vi "Pickering7.vi"(3 "Xmit Ring":i8=1) -> (0 "error out":errorcluster, 2 "dup VISA resource name":refnum<visa-resource-name>)   [LabVIEW 2022 SP3]
uses:
  Motion Controllers/-MotionRoutines/MotionGlobals.vi
panel:
  # "A zero clears all switches. 1-5 selects Xmit ring"
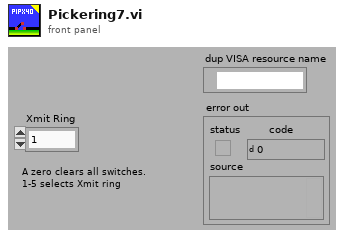
[diagram p1: front panel]
types:
  T1 = typedef "location.ctl" = enum16{"Automatic", "WCM Main", "Hawaii", "Columbia MM3000", "Columbia  NI System", "NYU", "RRI 2", "UHI Allen", "CUMC RT", "Chiba", "Stony Brook", "WCM Microscopy", "WCM Aeoretch", "WCM Optics Lab", "WCM Main 2Axis", "WCM Rotation", "WCM SAM SMAC", "SERI GP"}
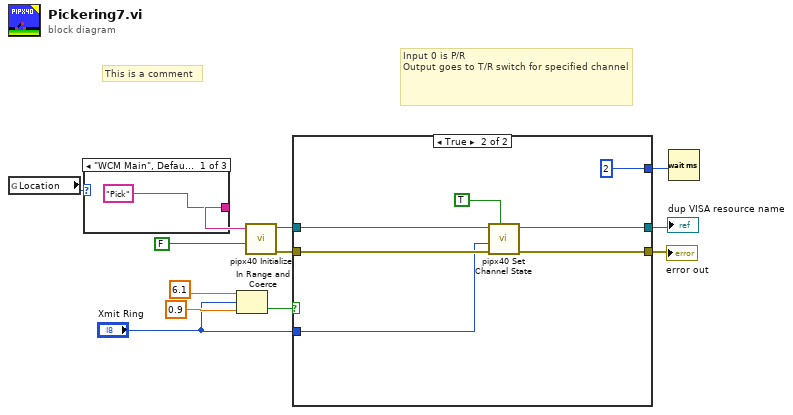
[diagram p0: block diagram]
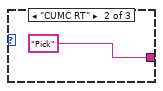
[diagram p2: hidden frame]
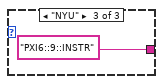
[diagram p3: hidden frame]
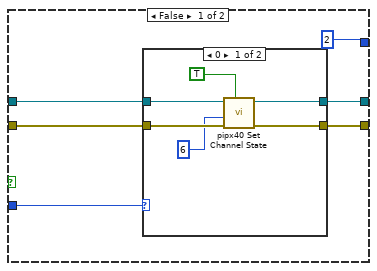
[diagram p4: hidden frame]
diagram:
  # "This is a comment"
  # "Input 0 is P/R\nOutput goes to T/R switch for specified channel"
  n1 = global read "MotionGlobals.vi" "Location"() -> (w2:T1)
  n2 = case shown="\"WCM Main\", Default" w2 {
    tunnel: ["Pick" ("VISA Resource Name") "Pick" ("VISA Resource Name") "PXI6::9::INSTR" ("VISA Resource Name")] -> w1
    frame "WCM Main", Default {
    }
    frame "CUMC RT" {
    }
    frame "NYU" {
    }
  }
  n3 = In Range and Coerce(upper limit=6.1, x="Xmit Ring", lower limit=0.9) -> (In Range?=w10:bool)  [unwired: 1 out]
  n4 = call <instrlib>:"pipx40 Initialize.vi"("reset device"=FALSE, "resource name"=w1) -> ("error out"=w5:errorcluster, "instrument handle out"=w6:refnum<visa-resource-name>)  [unwired: 8 in]
  n5 = case shown="True" w10 {
    tunnel: "Xmit Ring" -> [w21 w31]
    tunnel: [w20 w35] -> w8
    tunnel: [w19 w34] -> w7
    tunnel: w6 -> [w17 w36]
    tunnel: w5 -> [w18 w33]
    tunnel: [2 2] -> w3
    frame False {
      n6 = case shown="0" w21 {
        tunnel: [w25 w29] -> w20
        tunnel: [w24 w28] -> w19
        tunnel: w18 -> [w23 w28]
        tunnel: w17 -> [w26 w29]
        frame 0 {
          n7 = call <instrlib>:"pipx40 Set Channel State.vi"("action"=TRUE, "error in (no error)"=w23, "channel number"=6, "instrument handle"=w26) -> ("error out"=w24:errorcluster, "instrument handle out"=w25:refnum<visa-resource-name>)  [unwired: 6 in]
        }
        frame 1, Default {
        }
      }
    }
    frame True {
      (unwired) 10
      n8 = call <instrlib>:"pipx40 Set Channel State.vi"("action"=TRUE, "error in (no error)"=w33, "channel number"=w31, "instrument handle"=w36) -> ("error out"=w34:errorcluster, "instrument handle out"=w35:refnum<visa-resource-name>)  [unwired: 6 in]
    }
  }
  "dup VISA resource name" <- w8
  "error out" <- w7
  n9 = Wait (ms)(milliseconds to wait=w3) -> ()  [unwired: 1 out]
